vi "Send Update Energy Storage Parameter.vi"(7 "Message Priority (Normal)":T3=enum."Normal", 8 "error in":errorcluster, 10 "Energy Storage Parameters":T1, 11 "Message Enqueuer":refnum<class "Message Enqueuer.lvclass">) -> (0 "error out":errorcluster, 3 "Message Enqueuer out":refnum<class "Message Enqueuer.lvclass">)   [LabVIEW 2016, in "Optimization Framework.lvlib" / "Update Energy Storage Parameter Msg.lvclass"]
doc: "This VI sends the message to an actor."
uses:
  Update Energy Storage Parameter Msg.lvclass
  <vilib>/ActorFramework/Message Enqueuer/Message Enqueuer.lvclass
  <vilib>/ActorFramework/Message Enqueuer/Message Priority.ctl
  Optimization/Controls/Optimization Parameters Energy Storage.ctl
  Optimization/Controls/Device Control Capabilities.ctl
  C:/Program Files (x86)/National Instruments/LabVIEW 2016/vi.lib/ActorFramework/Message/Message.lvclass
  Update Energy Storage Parameter Msg.lvclass/Update Energy Storage Parameter Msg.ctl
  <vilib>/ActorFramework/Message Enqueuer/Message Enqueuer.lvclass/Message Enqueuer.ctl
  <vilib>/ActorFramework/Message Priority Queue/Priority Enqueue.vi
  Optimization/Optimization.lvclass
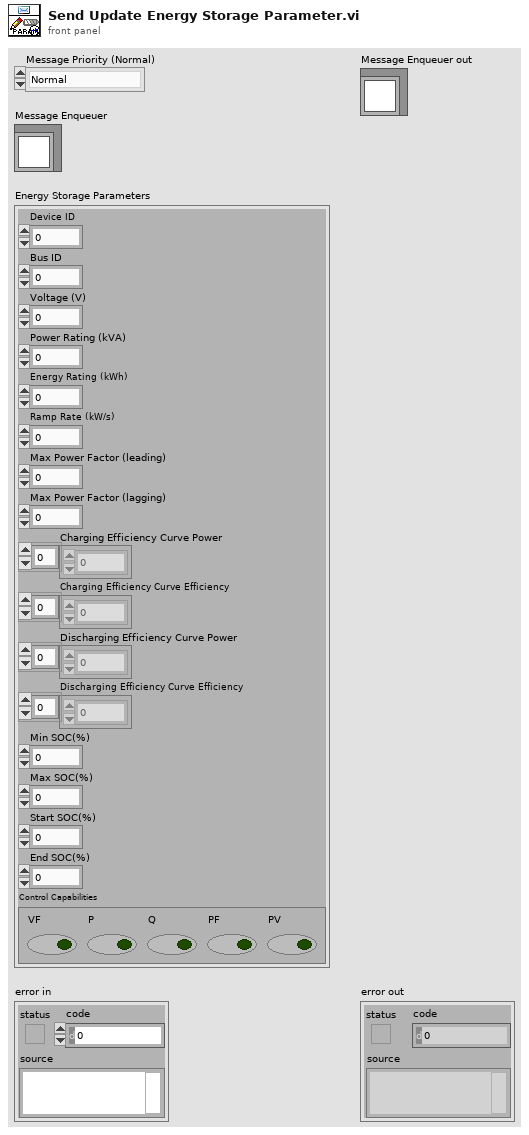
[diagram p1: front panel]
types:
  T1 = typedef "Optimization Framework.lvlib/Optimization.lvclass/Optimization Parameters Energy Storage.ctl" = cluster{"Device ID":u64, "Bus ID":u16, "Voltage (V)":dbl, "Power Rating (kVA)":dbl, "Energy Rating (kWh)":dbl, "Ramp Rate (kW/s)":dbl, "Max Power Factor (leading)":dbl, "Max Power Factor (lagging)":dbl, "Charging Efficiency Curve Power":dbl[], "Charging Efficiency Curve Efficiency":dbl[], "Discharging Efficiency Curve Power":dbl[], "Discharging Efficiency Curve Efficiency":dbl[], "Min SOC(%)":dbl, "Max SOC(%)":dbl, "Start SOC(%)":dbl, "End SOC(%)":dbl, "Control Capabilities":T2}
  T2 = typedef "Optimization Framework.lvlib/Optimization.lvclass/Device Control Capabilities.ctl" = cluster{"VF":bool, "P":bool, "Q":bool, "PF":bool, "PV":bool}
  T3 = typedef "Actor Framework.lvlib/Message Enqueuer.lvclass/Message Priority.ctl" = enum16{"Low", "Normal", "High"}
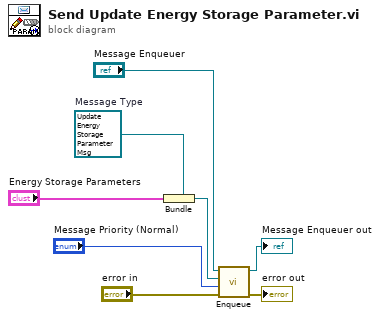
[diagram p0: block diagram]
diagram:
  w5 = refnum<class "Update Energy Storage Parameter Msg.lvclass"> refnum  # Message Type
  n1 = Bundle(cluster=w5, "Energy Storage Parameters") -> (w4:refnum<class "Update Energy Storage Parameter Msg.lvclass">)
  n2 = call <vilib>:"Enqueue.vi"("error in (no error)"="error in", "Message Priority (Normal)"="Message Priority (Normal)", "Message"=w4, "Message Enqueuer in"="Message Enqueuer") -> ("error out"=→"error out":errorcluster, "Message Enqueuer out"=→"Message Enqueuer out":refnum<class "Message Enqueuer.lvclass">)  [unwired: 6 in]
